vi "Word_Add_Document.vi"(0 "Word.Documents":refnum<k7>, 1 "document path":path, 2 "error in":errorcluster) -> (3 "Word._Document":refnum<k7>, 4 "Word.Tables":refnum<k7>, 5 "Word.InlineShapes":refnum<k7>, 6 "error out":errorcluster)   [LabVIEW 2010, in "NI_ReportGenerationToolkit.lvlib"]
uses:
  <vilib>/addons/_office/NI_ReportGenerationToolkit.lvlib
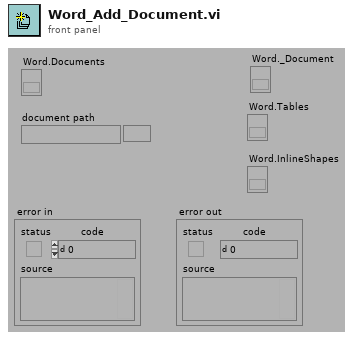
[diagram p1: front panel]
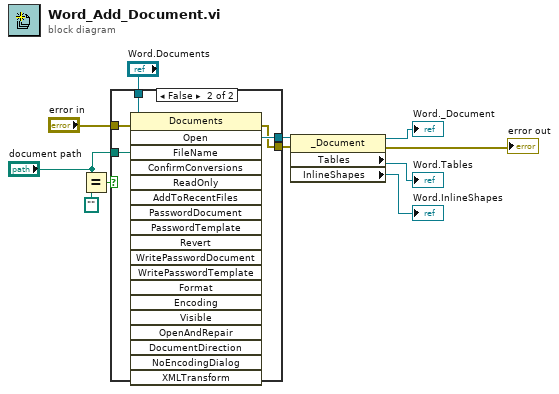
[diagram p0: block diagram]
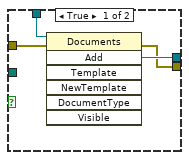
[diagram p2: hidden frame]
diagram:
  n1 = Equal?(x="document path", y=path "") -> (x = y?=w9:bool)
  n2 = case shown="False" w9 {
    tunnel: "Word.Documents" -> [w15 w20]
    tunnel: "error in" -> [w14 w19]
    tunnel: [w13 w18] -> w2
    tunnel: [w12 w17] -> w3
    tunnel: "document path" -> [_ w16]
    frame True {
      n3 = invoke class="Documents" method="Add"(reference=w15, error in=w14) -> (error out=w12:errorcluster, "Add"=w13:refnum<k7>)  [unwired: 5 in, 5 out]
    }
    frame False {
      n4 = invoke class="Documents" method="Open"(reference=w20, error in=w19, "FileName"=w16) -> (error out=w17:errorcluster, "Open"=w18:refnum<k7>)  [unwired: 16 in, 17 out]
    }
  }
  n5 = property class="_Document"(reference=w2, error in=w3) -> (reference out=→"Word._Document":refnum<k7>, error out=→"error out":errorcluster, "Tables"=→"Word.Tables":refnum<k7>, "InlineShapes"=→"Word.InlineShapes":refnum<k7>)
